vi "Display Logo.vi"(8 "error in":errorcluster) -> (0 "error out":errorcluster)   [LabVIEW 2013]
panel:
  in  "node":string
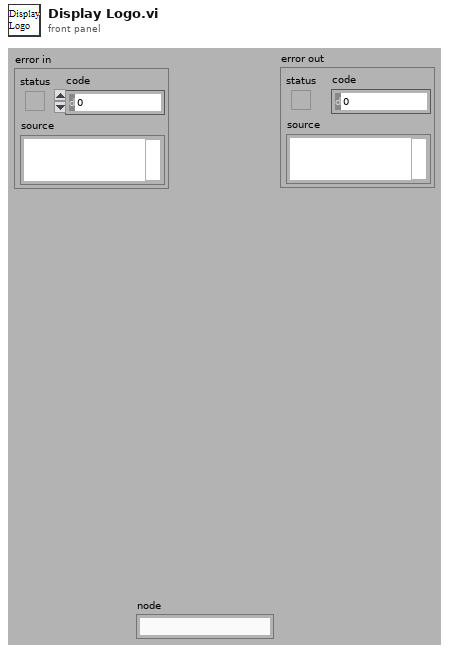
[diagram p1: front panel]
types:
  T1 = cluster{"Height":u32, "Width":u32, "is_bigendian?":u8, "Step":u32, "Data":u8[], "Encoding":string, "Frame ID":string}
  T2 = typedef "_ROSControl.ctl" = cluster{"topic port":u16, "Node":string, "topic":string, "type":string, "node port":u32, "error ":errorcluster, "Direction":T3, "APIs":string[]}
  T3 = typedef "_ROSDirection.ctl" = enum16{"Node", "Publisher", "Subscriber", "Service Client"}
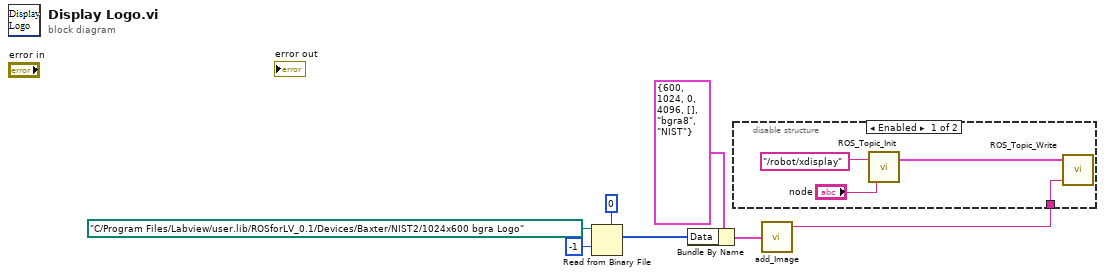
[diagram p0: block diagram]
diagram:
  n1 = Read from Binary File(5:u8 0, 10:-1 ("count (1)"), 11:path "C:/Program Files/Labview/user.lib/ROSforLV_0.1/Devices/Baxter/NIST2/1024x600 bgra Logo" ("file (use dialog)")) -> (2:w1:u8[])  [unwired: 3 in, 3 out]
  n2 = Bundle By Name(cluster=T1 {"Height"=600, "Width"=1024, "is_bigendian?"=0, "Step"=4096, "Data"=[], "Encoding"="bgra8", "Frame ID"="NIST"} ("ROS Image"), "Data"=w1) -> (w6:T1)
  n3 = call "add_Image.vi"("ROS Image"=w6) -> ("msg out"=w5:string)  [unwired: 4 in]
  n4 = disable-structure shown="Enabled" {
    disable-tunnel: w5 -> [w11 _]
    frame Enabled {
      n5 = call "ROS_Topic_Init.vi"("node"="node", "topic"="/robot/xdisplay") -> ("ROS out"=w8:T2)  [unwired: 1 in]
      n6 = call "ROS_Topic_Write.vi"("Msg in"=w11, "ROS in"=w8) -> ()  [unwired: 2 in, 1 out]
    }
    frame Disabled {
    }
  }
